vi "测试matlab文件读取训练模型.vi"() -> ()   [LabVIEW 2018]
panel:
  in  "Real 6":dbl
  in  "Real 5":dbl
  in  "Real 4":dbl
  in  "Real 3":dbl
  in  "停止":bool
  out "Real 2":dbl
  out "Real":dbl
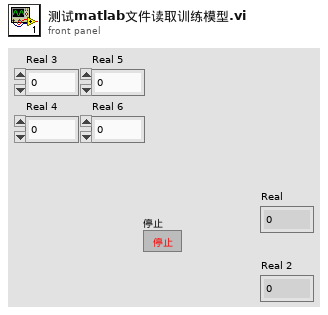
[diagram p1: front panel]
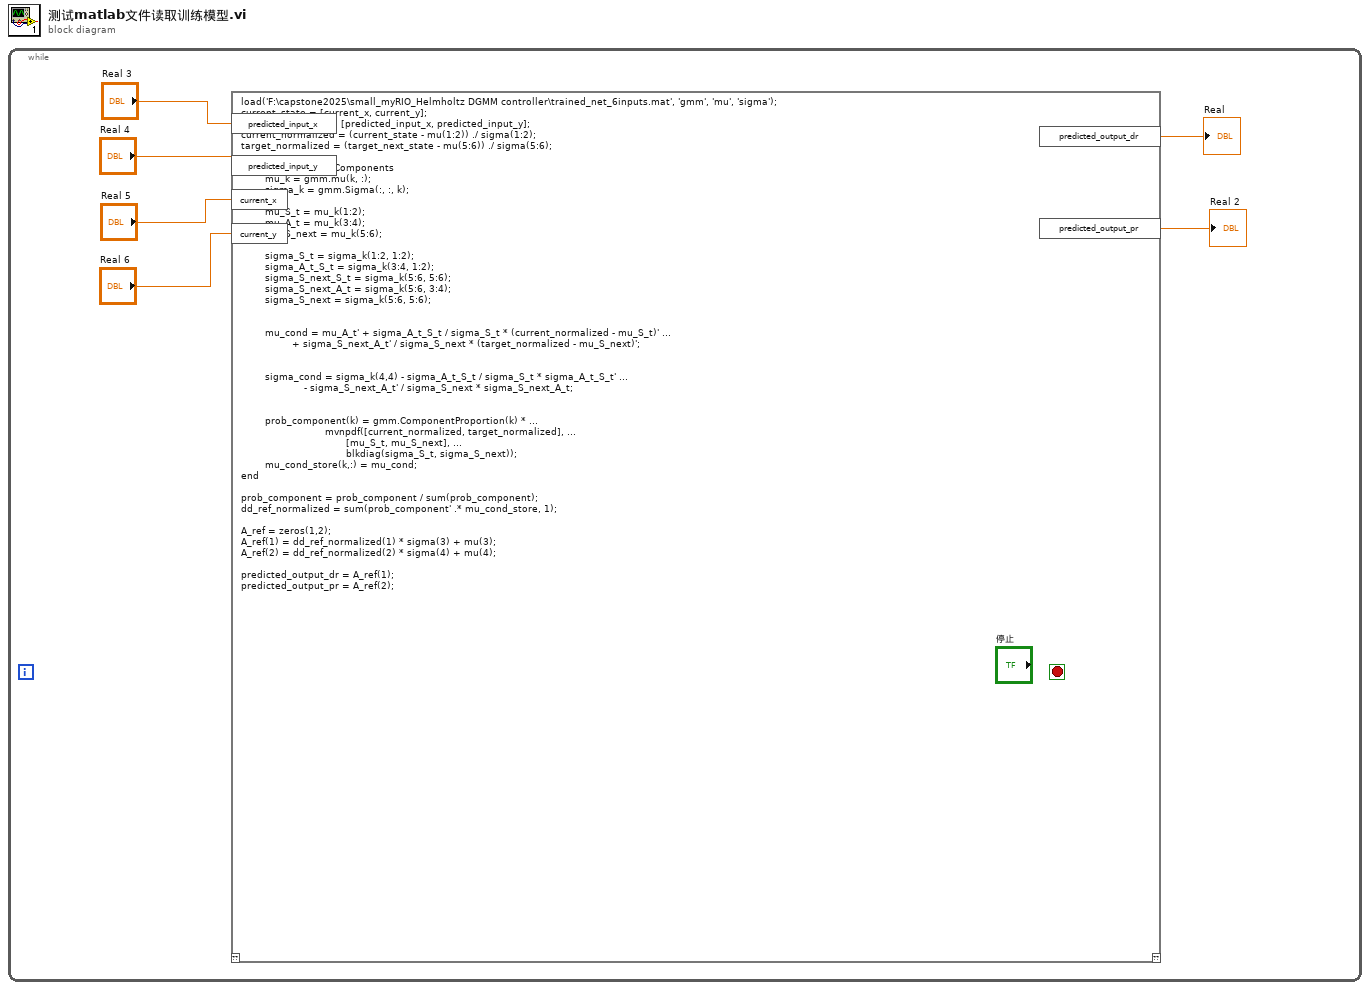
[diagram p0: block diagram]
diagram:
  n1 = while {
    stop <- "停止" stop-if-true
    n2 = script code="load('F:\\capstone2025\\small_myRIO_Helmholtz DGMM controller\\trained_net_6inputs.mat', 'gmm', 'mu', 'sigma');\ncurrent_state = [current_x, current_y];\ntarget_next_state = [predicted_input_x, predicted_input_y];\ncurrent_normalized = (current_state - mu(1:2)) ./ sigma(1:2);\ntarget_normalized = (target_next_state - mu(5:6)) ./ sigma(5:6);\n\nfor k = 1:gmm.NumComponents\n        mu_k = gmm.mu(k, :);           \n        sigma_k = gmm.Sigma(:, :, k);  \n        \n        mu_S_t = mu_k(1:2);       \n        mu_A_t = mu_k(3:4);         \n        mu_S_next = mu_k(5:6);   \n        \n        sigma_S_t = sigma_k(1:2, 1:2);\n        sigma_A_t_S_t = sigma_k(3:4, 1:2);\n        sigma_S_next_S_t = sigma_k(5:6, 5:6);\n        sigma_S_next_A_t = sigma_k(5:6, 3:4);\n        sigma_S_next = sigma_k(5:6, 5:6);\n        \n     \n        mu_cond = mu_A_t' + sigma_A_t_S_t / sigma_S_t * (current_normalized - mu_S_t)' ...\n                 + sigma_S_next_A_t' / sigma_S_next * (target_normalized - mu_S_next)';\n\n\n        sigma_cond = sigma_k(4,4) - sigma_A_t_S_t / sigma_S_t * sigma_A_t_S_t' ...\n                     - sigma_S_next_A_t' / sigma_S_next * sigma_S_next_A_t;\n        \n\n        prob_component(k) = gmm.ComponentProportion(k) * ...\n                            mvnpdf([current_normalized, target_normalized], ...\n                                   [mu_S_t, mu_S_next], ...\n                                   blkdiag(sigma_S_t, sigma_S_next));\n        mu_cond_store(k,:) = mu_cond;   \nend\n\nprob_component = prob_component / sum(prob_component);\ndd_ref_normalized = sum(prob_component' .* mu_cond_store, 1);\n\nA_ref = zeros(1,2);\nA_ref(1) = dd_ref_normalized(1) * sigma(3) + mu(3);\nA_ref(2) = dd_ref_normalized(2) * sigma(4) + mu(4);\n\npredicted_output_dr = A_ref(1);\npredicted_output_pr = A_ref(2);"("predicted_input_y"="Real 4", "predicted_input_x"="Real 3", "current_y"="Real 6", "current_x"="Real 5") -> ("predicted_output_dr"=→"Real":dbl, "predicted_output_pr"=→"Real 2":dbl)  [unwired: 1 in, 1 out]
  }
